vi "start_sweep.vi"(8 "error in (no error)":errorcluster, 11 "ScanModeDL091001Scaffold in":refnum<class "ImagingModeDL091001Scaffold.lvclass">) -> (0 "error out":errorcluster, 3 "ScanModeDL091001Scaffold out":refnum<class "ImagingModeDL091001Scaffold.lvclass">)   [LabVIEW 2010, in "ImagingModeDL091001Scaffold.lvclass"]
uses:
  ImagingModeDL091001Scaffold.lvclass
  ImagingModeDL090923Scaffold/ImagingModeDL090923Scaffold/ImagingModeDL090923Scaffold.lvclass
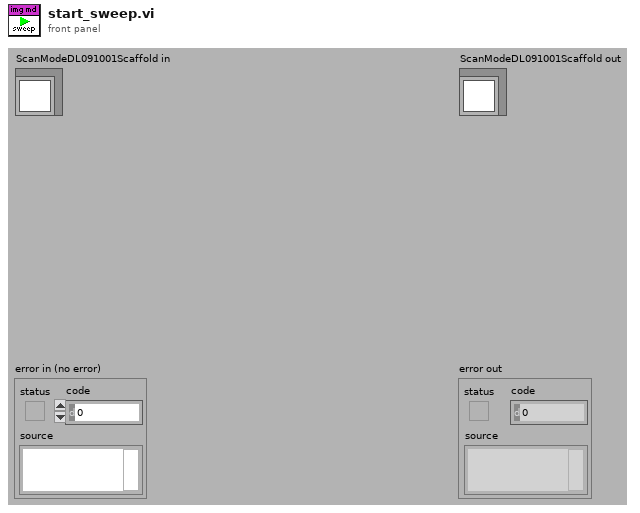
[diagram p1: front panel]
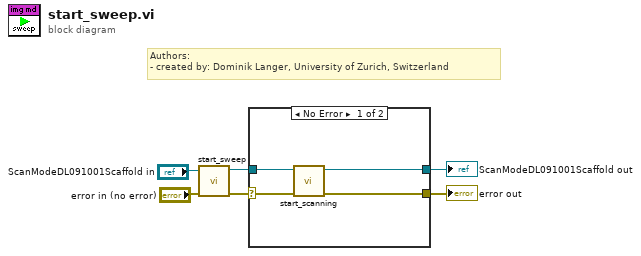
[diagram p0: block diagram]
diagram:
  # "Authors: \n- created by: Dominik Langer, University of Zurich, Switzerland"
  n1 = call-parent "start_sweep.vi"("error in (no error)"="error in (no error)", "ScanModeDL090923Scaffold in"="ScanModeDL091001Scaffold in") -> ("error out"=w3:errorcluster, "ScanModeDL090923Scaffold out"=w1:refnum<class "ImagingModeDL091001Scaffold.lvclass">)  [unwired: 8 in]
  n2 = case shown="No Error" w3 {
    selector: w3 -> [w7 w12]
    tunnel: [w10 w12] -> w6
    tunnel: [w8 w11] -> w5
    tunnel: w1 -> [w9 w11]
    frame No Error {
      n3 = call-dynamic "start_scanning.vi"("error in (no error)"=w7, "ScanModeDL090923Scaffold in"=w9) -> ("error out"=w10:errorcluster, "ScanModeDL090923Scaffold out"=w8:refnum<class "ImagingModeDL091001Scaffold.lvclass">)  [unwired: 8 in]
    }
    frame Error {
    }
  }
  "error out" <- w6
  "ScanModeDL091001Scaffold out" <- w5
